vi "ReadTemp.vi"() -> ()   [LabVIEW 2010]
uses:
  <vilib>/Instr/_visa.llb/VISA Configure Serial Port (Instr).vi
panel:
  out "error out":errorcluster
  out "Temp25Hz":dbl format="%#_3g"
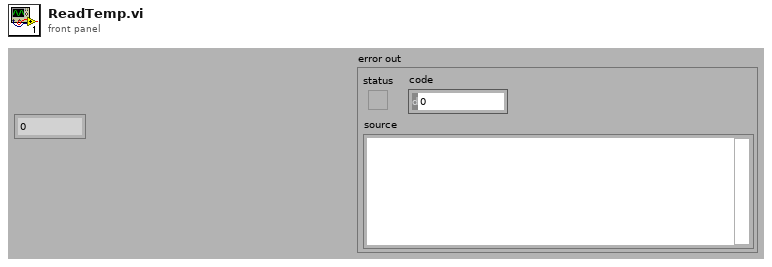
[diagram p1: front panel]
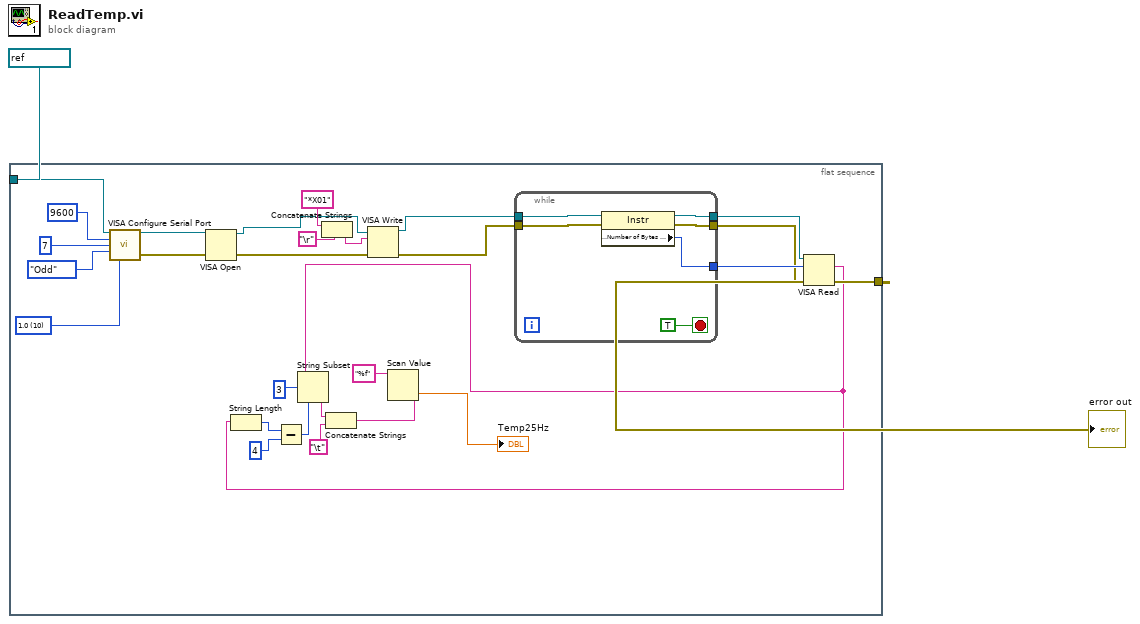
[diagram p0: block diagram]
diagram:
  n1 = flat-sequence {
    tunnel: refnum<visa-resource-name> "COM5" ("VISA Omega (Serial - COM1)") -> [w12]
    tunnel: [w11] -> w2
    frame #0 {
      w5 = u16 10 items=["1.0"=10, "1.5"=15, "2.0"=20] ("stop bits (10: 1 bit)")
      n2 = call-poly "VISA Configure Serial Port"("VISA resource name"=w12, "baud rate (9600)"=u32 9600, "data bits (8)"=u16 7, "parity (0:none)"=enum16{"None", "Odd", "Even", "Mark", "Space"}."Odd", "stop bits (10: 1 bit)"=w5) -> ("VISA resource name out"=w7:refnum<visa-resource-name>, "error out"=w15:errorcluster)  [unwired: 9 in]
      n3 = VISA Open(VISA resource name=w7) -> (VISA resource name=w6:refnum<visa-resource-name>)  [unwired: 4 in, 1 out]
      n4 = Concatenate Strings("*X01", "\r") -> (w18:string)
      n5 = VISA Write(VISA resource name=w6, write buffer=w18, error in (no error)=w15) -> (VISA resource name out=w29:refnum<visa-resource-name>, error out=w19:errorcluster)  [unwired: 1 out]
      n6 = while {
        tunnel: w29 -> [w35]
        tunnel: [w32] -> w21
        tunnel: [w34] -> w20
        tunnel: w19 -> [w33]
        tunnel: [w31] -> w8
        stop <- TRUE stop-if-true
        n7 = property class="Instr"(reference=w35, error in=w33) -> (reference out=w31:refnum<visa-resource-name>, error out=w34:errorcluster, "Serial Settings:Number of Bytes at Serial Port"=w32:u32)
      }
      n8 = VISA Read(VISA resource name=w8, byte count=w21, error in (no error)=w20) -> (read buffer=w22:string, error out=w11:errorcluster)  [unwired: 2 out]
      n9 = String Length(string=w22) -> (length=w24:i32)
      n10 = Subtract(x=w24, y=4) -> (x-y=w26:i32)
      n11 = String Subset(string=w22, offset (0)=3, length (rest)=w26) -> (substring=w27:string)
      n12 = Concatenate Strings(w27, "\t") -> (w13:string)
      n13 = Scan Value(string=w13, format string="%f") -> (value=→"Temp25Hz":dbl)  [unwired: 1 in, 1 out]
    }
  }
  "error out" <- w2
